vi "Add Monitor Recorders.vi"(6 "Reset":bool, 8 "error in (no error)":errorcluster, 10 "Module type":T1, 11 "Monitor-Pulse in":refnum<class "Monitor-Pulse.lvclass">) -> (0 "error out":errorcluster, 2 "Actot names out":string[](array[string]), 3 "Monitor-Pulse out":refnum<class "Monitor-Pulse.lvclass">)   [LabVIEW 2016, in "Monitor-Pulse.lvclass"]
uses:
  Monitor-Pulse.lvclass
  Module Types.ctl
  Instrument Actor/Instrument Actor.lvclass
  C:/github/Measure_core/Template Module/Template Module.lvclass
  Recorders/Micron Optics/Micron Optics Recorder.lvclass
  C:/github/Measure_core/Instrument Actor/Instrument Actor.lvclass
  NHMFL_Core/Libraries/Instruments/Micron Optics/Micron Hyperion Driver/Micron Hyperion Driver.lvclass
  C:/github/NHMFL_Core/Libraries/Instruments/Micron Optics/Micron Optics Driver/Micron Optics Driver.lvclass
  Spectrum Recorder too/Spectrum Recorder too.lvclass
  NHMFL_Core/Libraries/Red Pitaya/RP Core/Red Pitaya Transceiver Driver/Red Pitaya Transceiver Driver.lvclass
  C:/github/NHMFL_Core/Libraries/Instruments/Instrument Driver/Instrument Driver.lvclass
  Instrument Actor/Instrument Actor.lvclass/Instrument Actor.ctl
  Monitor-Pulse.lvclass/Monitor-Pulse.ctl
  Instrument Actor/Write Instrument driver.vi
  Recorders/Micron Optics/Write Micron Optics Driver.vi
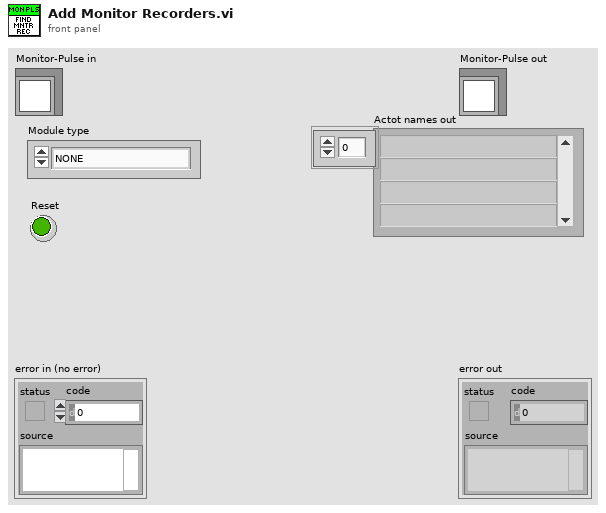
[diagram p1: front panel]
types:
  T1 = typedef "Module Types.ctl" = enum16{"NONE", "NI-DAQmx", "NI-Scope", "Red Pitaya Digitizer", "GaGe", "VISA Device", "Red Pitaya Lockin", "Monitor Controller", "Pulse Controller", "Integrate Pulse", "Lockin Processor", "File converter", "NHMFL Synthesizer", "Micron Hyperion", "Spectrum Recorder"}
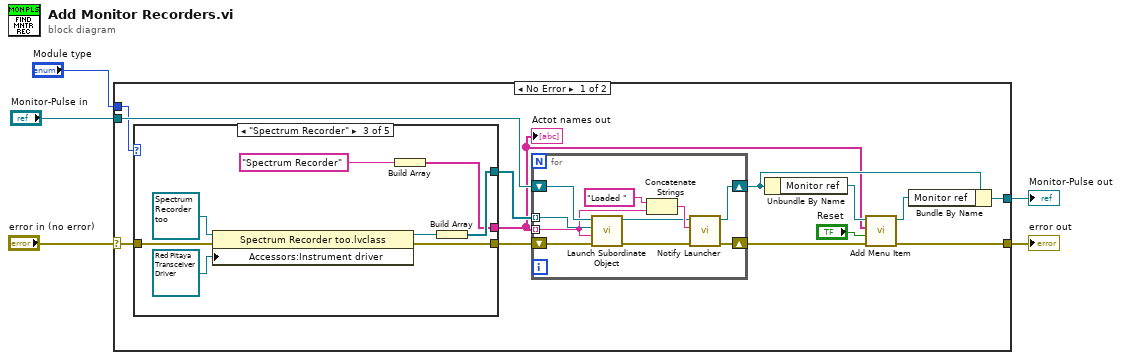
[diagram p0: block diagram]
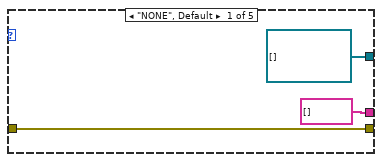
[diagram p2: hidden frame]
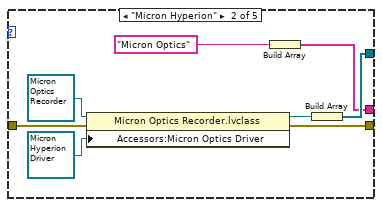
[diagram p3: hidden frame]
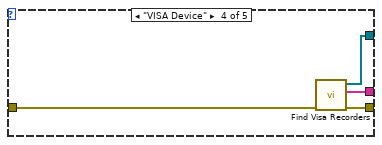
[diagram p4: hidden frame]
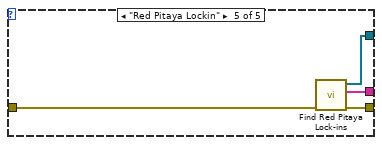
[diagram p5: hidden frame]
diagram:
  n1 = case shown="No Error" "error in (no error)" {
    selector: "error in (no error)" -> [w18 w57]
    tunnel: [w7 w57] -> w4
    tunnel: [w8 w56] -> w2
    tunnel: "Monitor-Pulse in" -> [w17 w56]
    tunnel: "Module type" -> [w14 _]
    frame No Error {
      n2 = case shown="\"Spectrum Recorder\"" w14 {
        tunnel: w18 -> [w19 w28 w36 w41 w44]
        tunnel: [refnum<class "Instrument Actor.lvclass">[] [] ("Recorders List") w29 w37 w40 w43] -> w16
        tunnel: [string[] [] ("Names") w22 w30 w39 w42] -> w10
        tunnel: [w19 w27 w35 w38 w45] -> w15
        frame "NONE", Default {
        }
        frame "Micron Hyperion" {
          n3 = property class="Micron Optics Recorder.lvclass"(reference=refnum<class "Micron Optics Recorder.lvclass"> refnum ("Micron Optics Recorder.lvclass"), error in=w28, "Accessors:Micron Optics Driver"=refnum<class "Micron Hyperion Driver.lvclass"> refnum ("Micron Hyperion Driver.lvclass")) -> (reference out=w25:refnum<class "Micron Optics Recorder.lvclass">, error out=w27:errorcluster)
          n4 = Build Array("Micron Optics") -> (w22:string[])
          n5 = Build Array(w25) -> (w29:refnum<class "Micron Optics Recorder.lvclass">[])
        }
        frame "Spectrum Recorder" {
          n6 = property class="Spectrum Recorder too.lvclass"(reference=refnum<class "Spectrum Recorder too.lvclass"> refnum ("Spectrum Recorder too.lvclass"), error in=w36, "Accessors:Instrument driver"=refnum<class "Red Pitaya Transceiver Driver.lvclass"> refnum ("Red Pitaya Transceiver Driver.lvclass")) -> (reference out=w33:refnum<class "Spectrum Recorder too.lvclass">, error out=w35:errorcluster)
          n7 = Build Array("Spectrum Recorder") -> (w30:string[])
          n8 = Build Array(w33) -> (w37:refnum<class "Spectrum Recorder too.lvclass">[])
        }
        frame "VISA Device" {
          n9 = call "Find Visa Recorders.vi"("Error In"=w41) -> ("Error Out"=w38:errorcluster, "Names"=w39:string[], "Recorders List"=w40:refnum<class "Instrument Actor.lvclass">[])  [unwired: 8 in]
        }
        frame "Red Pitaya Lockin" {
          n10 = call "Find Red Pitaya Lock-ins.vi"("Error In"=w44) -> ("Error Out"=w45:errorcluster, "Names"=w42:string[], "Instruments out"=w43:refnum<class "Instrument Actor.lvclass">[])  [unwired: 7 in, 1 out]
        }
      }
      "Actot names out" <- w10
      n11 = for {
        shift-right: [w49] -> w11
        shift-left: w17 -> [w55]
        shift-right: [w47] -> w9
        shift-left: w15 -> [w54]
        tunnel: w16 -> [w53] mode=indexing
        tunnel: w10 -> [w46] mode=indexing
        n12 = call-dynamic "Launch Subordinate Object.vi"("error in (no error)"=w54, "Name"=w46, "Subordinate Object"=w53, "Measure Object in"=w55) -> ("error out"=w48:errorcluster, "Measure Object out"=w50:refnum<class "Monitor-Pulse.lvclass">)  [unwired: 5 in, 1 out]
        n13 = Concatenate Strings("Loaded " ("string"), w46) -> (w51:string)
        n14 = call-dynamic "Notify Launcher.vi"("error in (no error)"=w48, "Notification"=w51, "Application Controller in"=w50) -> ("error out"=w47:errorcluster, "Application Controller out"=w49:refnum<class "Monitor-Pulse.lvclass">)  [unwired: 7 in]
      }
      n15 = Unbundle By Name(w11) -> ("Monitor ref"=w12:refnum<vi>)
      n16 = call "Add Menu Item.vi"("error in (no error)"=w9, "Reset"="Reset", "Item Names"=w10, "Queed Listbox ref"=w12) -> ("error out"=w7:errorcluster, "Queed Listbox ref out"=w13:refnum<vi>)  [unwired: 5 in, 1 out]
      n17 = Bundle By Name(cluster=w11, "Monitor ref"=w13) -> (w8:refnum<class "Monitor-Pulse.lvclass">)
    }
    frame Error {
    }
  }
  "error out" <- w4
  "Monitor-Pulse out" <- w2
